vi "svfa_Average Array with Avg Checks (real) No State.vi"(0 "spectrum":dbl[](array[numeric]) format="%.2f", 1 "processing control":T1(ring), 7 "averaging parameters":T3={"averaging mode"=enum."No averaging", "weighting mode"=enum."Linear", "number of averages"=10, "linear mode"=enum."Auto restart"}, 11 "error in":errorcluster, 12 "averaging state info":T2={"complex FFT"=[], "real FFT"=[], "f0"=0.0, "df"=0.0, "averages completed"=0.0, "averaging parameters"={"averaging mode"=enum."No averaging", "weighting mode"=enum."Linear", "number of averages"=10, "linear mode"=enum."Auto restart"}} {"averages completed" format="%.2f"; "df" format="%.2f"; "f0" format="%.2f"; "real FFT" format="%.2f"; "complex FFT" format="%.2f"}) -> (4 "avg spectrum":dbl[](array[numeric]) format="%.2f", 6 "new spectrum ready":bool, 8 "averaging done":bool, 10 "averages completed":dbl, 14 "averaging state info":T2={"complex FFT"=[], "real FFT"=[], "f0"=0.0, "df"=0.0, "averages completed"=0.0, "averaging parameters"={"averaging mode"=enum."No averaging", "weighting mode"=enum."Linear", "number of averages"=10, "linear mode"=enum."Auto restart"}} {"averages completed" format="%.2f"; "df" format="%.2f"; "f0" format="%.2f"; "real FFT" format="%.2f"; "complex FFT" format="%.2f"}, 15 "error out":errorcluster)   [LabVIEW 2017]
uses:
  <vilib>/addons/_NISVFA/_Shared subVIs/Spectrum Averaging/svfa_No Average Array (real).vi
  <vilib>/addons/_NISVFA/_Shared subVIs/Spectrum Averaging/svfa_Average Array (real).vi
  <vilib>/addons/_NISVFA/_Shared subVIs/Spectrum Averaging/svfa_Peak Hold Array.vi
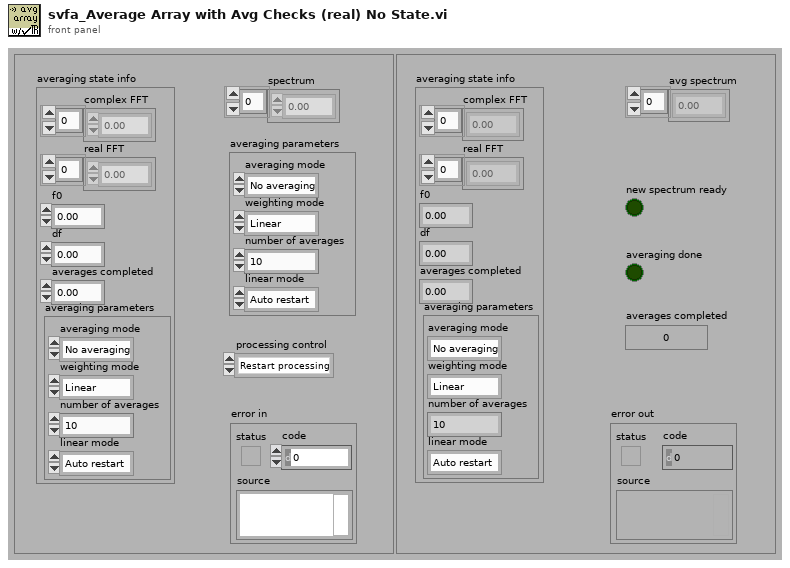
[diagram p1: front panel]
types:
  T1 = enum16{"Restart processing", "Continue processing", "Skip processing"}
  T2 = cluster{"complex FFT":cdb[], "real FFT":dbl[], "f0":dbl, "df":dbl, "averages completed":dbl, "averaging parameters":cluster{"averaging mode":enum16{"No averaging", "Vector averaging", "RMS averaging", "Peak hold"}, "weighting mode":enum16{"Linear", "Exponential"}, "number of averages":u32, "linear mode":enum16{"One shot", "Auto restart"}}}
  T3 = cluster{"averaging mode":enum16{"No averaging", "Vector averaging", "RMS averaging", "Peak hold"}, "weighting mode":enum16{"Linear", "Exponential"}, "number of averages":u32, "linear mode":enum16{"One shot", "Auto restart"}}
  T4 = cluster{"complex FFT":cdb[], "Mag/Real FFT":dbl[], "f0":dbl, "df":dbl, "averages completed":dbl, "averaging parameters":cluster{"averaging mode":enum16{"No averaging", "Vector averaging", "RMS averaging", "Peak hold"}, "weighting mode":enum16{"Linear", "Exponential"}, "number of averages":u32, "linear mode":enum16{"One shot", "Auto restart"}}}
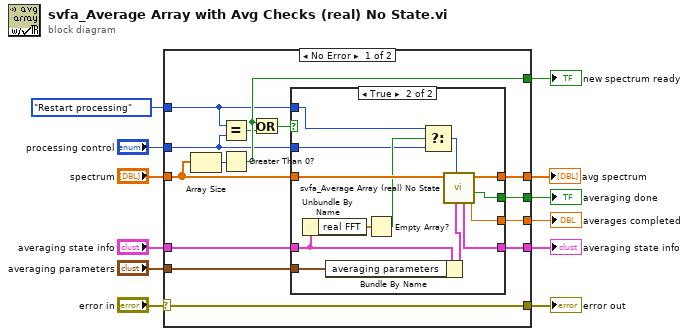
[diagram p0: block diagram]
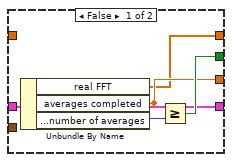
[diagram p2: hidden frame]
diagram:
  n1 = case shown="No Error" "error in" {
    selector: "error in" -> [w15 w45]
    tunnel: "spectrum" -> [w17 _]
    tunnel: [w25 w46] -> w11
    tunnel: [w23 _] -> w10
    tunnel: "averaging state info" -> [w22 w46]
    tunnel: "processing control" -> [w21 _]
    tunnel: [w19 _] -> w8
    tunnel: [w18 _] -> w7
    tunnel: "averaging parameters" -> [w13 _]
    tunnel: [w15 w45] -> w4
    tunnel: [w16 _] -> w3
    tunnel: T1."Restart processing" ("processing control") -> [w14 _]
    frame No Error {
      n2 = Array Size(array=w17) -> (size(s)=w26:i32)
      n3 = Equal?(x=w14, y=w21) -> (x = y?=w20:bool)
      n4 = Greater Than 0?(x=w26) -> (x > 0?=w23:bool)
      n5 = Or(x=w23, y=w20) -> (x .or. y?=w24:bool)
      n6 = case shown="True" w24 {
        tunnel: [w28 w43] -> w16
        tunnel: [w29 w40] -> w19
        tunnel: w22 -> [w30 w34]
        tunnel: [w30 w44] -> w25
        tunnel: w21 -> [_ w37]
        tunnel: [w31 w42] -> w18
        tunnel: w17 -> [_ w41]
        tunnel: w14 -> [_ w35]
        tunnel: w13 -> [_ w32]
        frame False {
          n7 = Unbundle By Name(w30) -> ("real FFT"=w28:dbl[], "averages completed"=w29:dbl, "averaging parameters.number of averages"=w27:u32)
          n8 = Greater Or Equal?(x=w29, y=w27) -> (x >= y?=w31:bool)
        }
        frame True {
          n9 = Unbundle By Name(w34) -> ("real FFT"=w39:dbl[])
          n10 = Bundle By Name(cluster=w34, "averaging parameters"=w32) -> (w33:T2)
          n11 = Empty Array?(array=w39) -> (empty?=w38:bool)
          n12 = Select(t=w35, s=w38, f=w37) -> (s? t:f=w36:T1)
          n13 = call <vilib>:"svfa_Average Array (real) No State.vi"("averaging state info in"=w33, "processing control"=w36, "array"=w41) -> ("averages completed"=w40:dbl, "averaging done"=w42:bool, "average array"=w43:dbl[], "averaging state info out"=w44:T4)  [unwired: 5 in]
        }
      }
    }
    frame Error {
    }
  }
  "avg spectrum" <- w3
  "averaging state info" <- w11
  "averages completed" <- w8
  "new spectrum ready" <- w10
  "averaging done" <- w7
  "error out" <- w4
